vi "Mouse Up (Deprecated).vi"(7 "Map Model in":refnum<class "Map Model.lvclass">, 8 "error in (no error)":errorcluster, 10 "Position":T1, 11 "Eraser in":refnum<class "Eraser.lvclass">) -> (0 "error out":errorcluster, 3 "Eraser out":refnum<class "Eraser.lvclass">, 5 "Map Model out":refnum<class "Map Model.lvclass">)   [LabVIEW 2020, in "Map Model.lvlib" / "Eraser.lvclass"]
uses:
  Eraser.lvclass
  <vilib>/Utility/miscctls.llb/LVPoint32TypeDef.ctl
  Map Model/Map Model.lvclass
  Undoable Tool/Undoable Tool.lvclass
  Tool/Tool.lvclass
  E:/Project/Labview-Projects/Completed projects/Map Editor/Models/Map Model/Tools/Undoable Tool/Undoable Tool.lvclass
  E:/Project/Labview-Projects/Completed projects/Map Editor/Models/Map Model/Tools/Tool/Tool.lvclass
panel:
  # "NOTICE -- YOU MUST LEAVE THIS NOTICE IN PLACE.\n\nCopyright (c) 2017, LIANG LIU Shawn.Liu.cn@gmail.com\nAll rights reserved.\n\nRedistribution and use in source and binary forms, with or without modification, are permitted provided that the following conditions are met:\n-Redistributions of source code must retain the above copyright notice, this list of conditions and the following disclaimer.\n-Redistributions in binary form must reproduce the above copyright notice, this list of conditions and the following disclaimer in the documentation and/or other materials provided with the distribution.\n-Neither the name of the eLp nor the names of its contributors may be used to endorse or promote products derived from this software without specific prior written permission.\n\nTHIS SOFTWARE IS PROVIDED BY THE COPYRIGHT HOLDERS AND CONTRIBUTORS \"AS IS\" AND ANY EXPRESS OR IMPLIED WARRANTIES, INCLUDING, BUT NOT LIMITED TO, THE IMPLIED WARRANTIES OF MERCHANTABILITY AND FITNESS FOR A PARTICULAR PURPOSE ARE DISCLAIMED. IN NO EVENT SHALL THE COPYRIGHT HOLDER OR CONTRIBUTORS BE LIABLE FOR ANY DIRECT, INDIRECT, INCIDENTAL, SPECIAL, EXEMPLARY, OR CONSEQUENTIAL DAMAGES (INCLUDING, BUT NOT LIMITED TO, PROCUREMENT OF SUBSTITUTE GOODS OR SERVICES; LOSS OF USE, DATA, OR PROFITS; OR BUSINESS INTERRUPTION) HOWEVER CAUSED AND ON ANY THEORY OF LIABILITY, WHETHER IN CONTRACT, STRICT LIABILITY, OR TORT (INCLUDING NEGLIGENCE OR OTHERWISE) ARISING IN ANY WAY OUT OF THE USE OF THIS SOFTWARE, EVEN IF ADVISED OF THE POSSIBILITY OF SUCH DAMAGE."
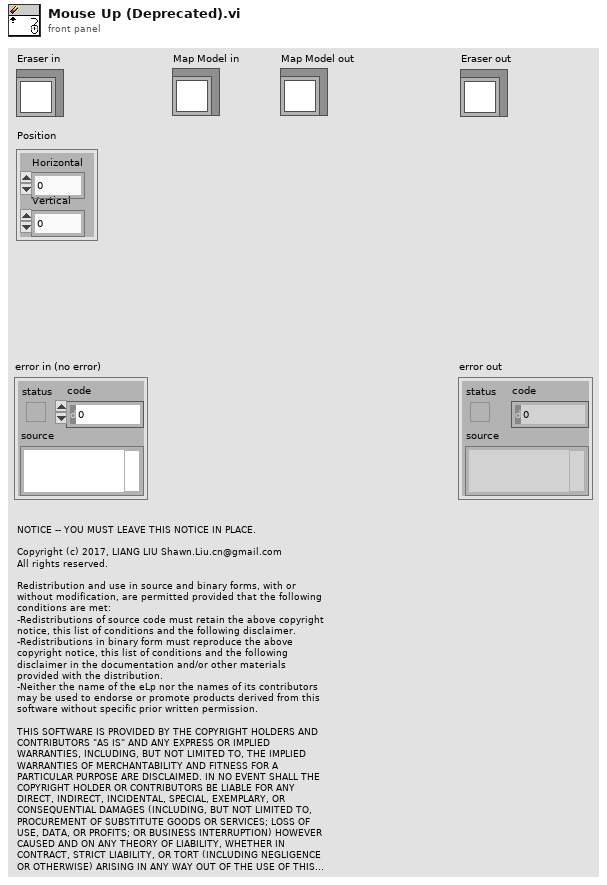
[diagram p1: front panel]
types:
  T1 = typedef "LVPoint32TypeDef.ctl" = cluster{"Horizontal":i32, "Vertical":i32}
  T2 = cluster{"Occupied Color":cluster{"Value":u8, "Color":u32}, "Free Color":cluster{"Value":u8, "Color":u32}, "Unknown Color":cluster{"Value":u8, "Color":u32}}
  T3 = typedef "imagedata.ctl" = cluster{"image type":i32, "image depth":i32, "image":u8[], "mask":u8[], "colors":u32[], "Rectangle":cluster{"left":i16, "top":i16, "right":i16, "bottom":i16}}
  T4 = cluster{"left":i16, "top":i16, "right":i16, "bottom":i16}
  T5 = typedef "LVPointTypeDef.ctl" = cluster{"Horizontal":i16, "Vertical":i16}
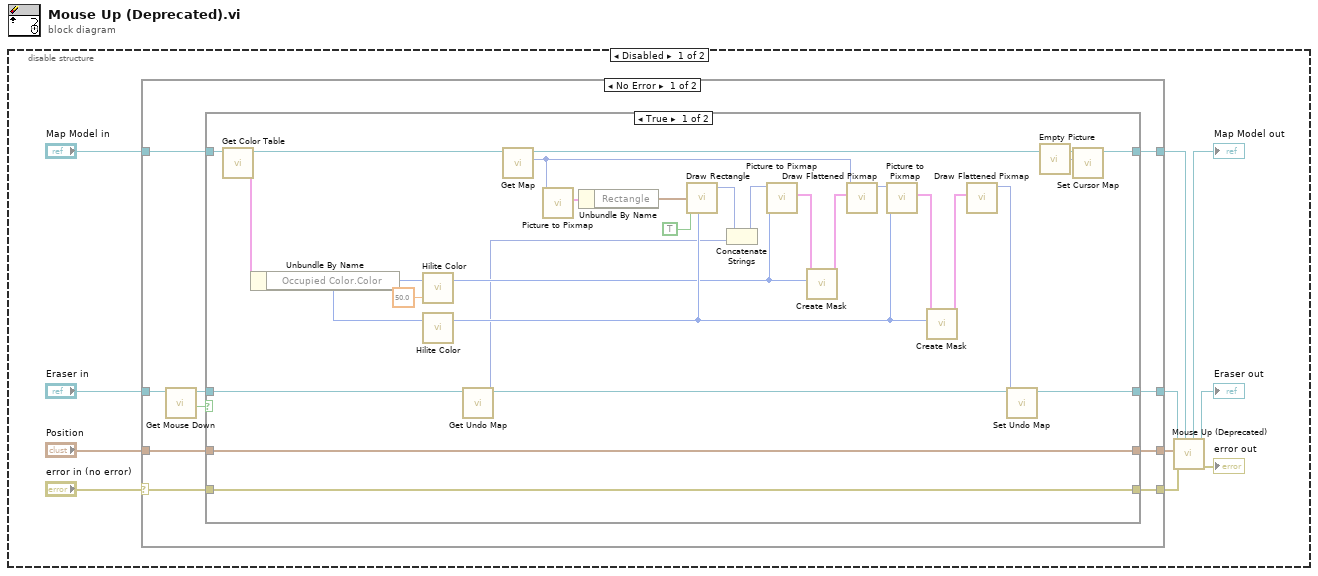
[diagram p0: block diagram]
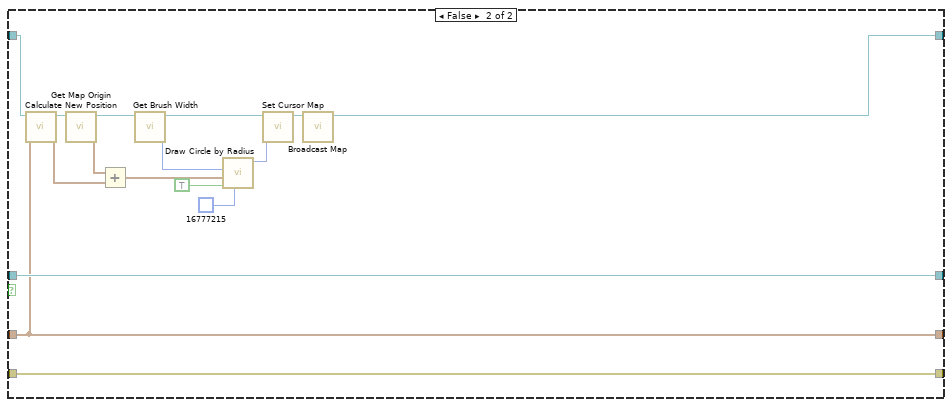
[diagram p2: hidden frame]
diagram:
  n1 = disable-structure shown="Disabled" {
    frame Disabled {
      n2 = case shown="No Error" "error in (no error)" {
        selector: "error in (no error)" -> [w18 w69]
        tunnel: "Map Model in" -> [w21 w68]
        tunnel: "Eraser in" -> [w20 w67]
        tunnel: "Position" -> [w19 w66]
        tunnel: [w17 w66] -> w5
        tunnel: [w16 w68] -> w3
        tunnel: [w15 w67] -> w2
        tunnel: [w14 w69] -> w1
        frame No Error {
          n3 = call "Get Mouse Down.vi"("Tool in"=w20) -> ("Mouse Down"=w12:bool, "Tool out"=w13:refnum<class "Eraser.lvclass">)  [unwired: 9 in]
          n4 = case shown="True" w12 {
            tunnel: w13 -> [w49 w63]
            tunnel: w21 -> [w48 w65]
            tunnel: [w23 w62] -> w16
            tunnel: [w42 w63] -> w15
            tunnel: w19 -> [w44 w51]
            tunnel: [w44 w51] -> w17
            tunnel: w18 -> [w46 w59]
            tunnel: [w46 w59] -> w14
            frame True {
              n5 = call "Get Color Table.vi"("Map Model in"=w48) -> ("Color Table"=w47:T2, "Map Model out"=w25:refnum<class "Map Model.lvclass">)  [unwired: 9 in]
              n6 = Unbundle By Name(w47) -> ("Occupied Color.Color"=w32:u32)
              n7 = call <vilib>:"Hilite Color.vi"("Percentage(30)"=50.0, "Color In"=w32) -> ("Hilite"=w29:u32)  [unwired: 1 out]
              n8 = call <vilib>:"Hilite Color.vi"("Color In"=w32) -> ("Hilite"=w31:u32)  [unwired: 1 in, 1 out]
              n9 = call "Get Undo Map.vi"("Undoable Tool in"=w49) -> ("Undo Map"=w26:picture, "Undoable Tool out"=w43:refnum<class "Eraser.lvclass">)  [unwired: 9 in]
              n10 = call "Get Map.vi"("Map Model in"=w25) -> ("Map"=w27:picture, "Map Model out"=w41:refnum<class "Map Model.lvclass">)  [unwired: 9 in]
              n11 = call <vilib>:"Picture to Pixmap.vi"("picture"=w27) -> ("image data"=w40:T3)  [unwired: 9 in, 1 out]
              n12 = Unbundle By Name(w40) -> ("Rectangle"=w39:T4)
              n13 = call <vilib>:"Draw Rectangle.vi"("rect"=w39, "fill?(F)"=TRUE, "color(black)"=w31) -> ("new picture"=w38:picture)  [unwired: 6 in]
              n14 = Concatenate Strings(w38, w26) -> (w30:picture)
              n15 = call <vilib>:"Picture to Pixmap.vi"("Background Color"=w29, "picture"=w30) -> ("image data"=w37:T3)  [unwired: 8 in, 1 out]
              n16 = call <vilib>:"Create Mask.vi"("Mask Color (Black)"=w29, "image data"=w37) -> ("image data"=w36:T3)  [unwired: 9 in]
              n17 = call <vilib>:"Draw Flattened Pixmap.vi"("image data"=w36, "picture"=w27) -> ("new picture"=w33:picture)  [unwired: 7 in]
              n18 = call <vilib>:"Picture to Pixmap.vi"("Background Color"=w31, "picture"=w33) -> ("image data"=w34:T3)  [unwired: 8 in, 1 out]
              n19 = call <vilib>:"Create Mask.vi"("Mask Color (Black)"=w31, "image data"=w34) -> ("image data"=w35:T3)  [unwired: 9 in]
              n20 = call <vilib>:"Draw Flattened Pixmap.vi"("image data"=w35) -> ("new picture"=w24:picture)  [unwired: 8 in]
              n21 = call "Set Undo Map.vi"("Undo Map"=w24, "Undoable Tool in"=w43) -> ("Undoable Tool out"=w42:refnum<class "Eraser.lvclass">)  [unwired: 9 in]
              n22 = call "Empty Picture"() -> ("empty picture"=w22:picture)
              n23 = call "Set Cursor Map.vi"("Cursor Map"=w22, "Map Model in"=w41) -> ("Map Model out"=w23:refnum<class "Map Model.lvclass">)  [unwired: 9 in]
            }
            frame False {
              n24 = call "Calculate New Position.vi"("Position in"=w51, "Map Model in"=w65) -> ("Position out"=w50:T1, "Map Model out"=w52:refnum<class "Map Model.lvclass">)  [unwired: 8 in]
              n25 = call "Get Map Origin.vi"("Map Model in"=w52) -> ("Map Origin"=w54:T5, "Map Model out"=w55:refnum<class "Map Model.lvclass">)  [unwired: 9 in]
              n26 = Add(x=w54, y=w50) -> (x+y=w53:T1)
              n27 = call "Get Brush Width.vi"("Map Model in"=w55) -> ("Brush Width"=w57:i32, "Map Model out"=w58:refnum<class "Map Model.lvclass">)  [unwired: 9 in]
              n28 = call <vilib>:"Draw Circle by Radius.vi"("color(black)"=u32 16777215, "fill?(F)"=TRUE, "pixel center"=w53, "radius"=w57) -> ("new picture"=w61:picture)  [unwired: 7 in]
              n29 = call "Set Cursor Map.vi"("Cursor Map"=w61, "Map Model in"=w58) -> ("Map Model out"=w64:refnum<class "Map Model.lvclass">)  [unwired: 9 in]
              n30 = call "Broadcast Map.vi"("Map Model in"=w64) -> ("Map Model out"=w62:refnum<class "Map Model.lvclass">)  [unwired: 9 in, 1 out]
            }
          }
        }
        frame Error {
        }
      }
      n31 = call-parent "Mouse Up (Deprecated).vi"("Map Model in"=w3, "error in (no error)"=w1, "Position"=w5, "Undoable Tool in"=w2) -> ("error out"=→"error out":errorcluster, "Undoable Tool out"=→"Eraser out":refnum<class "Eraser.lvclass">, "Map Model out"=→"Map Model out":refnum<class "Map Model.lvclass">)  [unwired: 5 in]
    }
    frame Enabled {
    }
  }
